vi "LS4 MoveAbsSingleAxis_SD.vi"(1 "Wait":bool=TRUE, 2 "Value":dbl format="%.2f", 3 "Axis":i32=1) -> (0 "Command executed":bool)   [LabVIEW 2015]
doc: "Move a single axis to the specified position. (1..4)\nIf 'Wait' is set to 'true', the VI waits till the position is reached."
uses:
  DLL/LStep4.dll
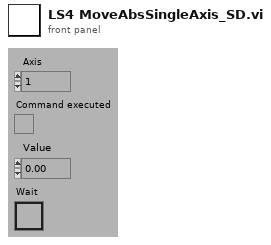
[diagram p1: front panel]
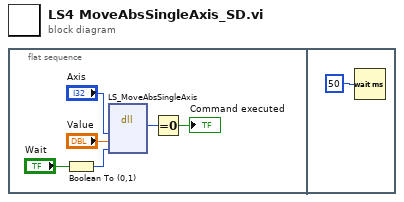
[diagram p0: block diagram]
diagram:
  n1 = flat-sequence {
    frame #0 {
      n2 = Boolean To (0,1)(Boolean="Wait") -> (0, 1=w2:i16)
      n3 = dll-call lib="G:/SD/TRANCON/DLL/LStep4.dll" fn="LS_MoveAbsSingleAxis"("Axis"="Axis", "Value"="Value", "Wait"=w2) -> ("type de retour"=w4:i32)  [unwired: 6 in, 2 out]
      n4 = Equal To 0?(x=w4) -> (x = 0?=→"Command executed":bool)
    }
    frame #1 {
      n5 = Wait (ms)(milliseconds to wait=u32 50) -> ()  [unwired: 1 out]
    }
  }
